vi "Write ItemID.vi"(8 "error in (no error)":errorcluster, 10 "ItemID":string, 11 "Standard VI Type in":refnum<class "Standard VI Type.lvclass">) -> (0 "error out":errorcluster, 3 "Standard VI Type out":refnum<class "Standard VI Type.lvclass">)   [LabVIEW 2020]
doc: "Basic write acceessor."
uses:
  Standard VI Type.lvclass
  Standard VI Type.lvclass/Standard VI Type.ctl
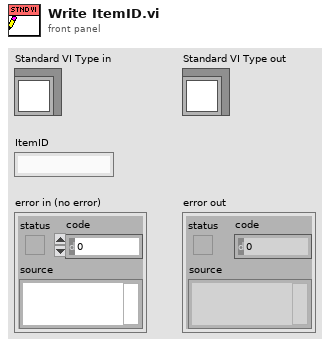
[diagram p1: front panel]
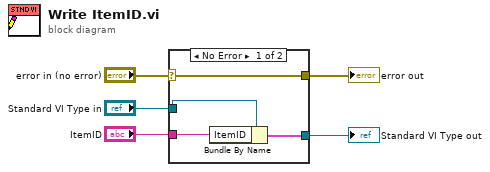
[diagram p0: block diagram]
diagram:
  n1 = case shown="No Error" "error in (no error)" {
    selector: "error in (no error)" -> [w9 w10]
    tunnel: [w9 w10] -> w4
    tunnel: [w7 w11] -> w2
    tunnel: "Standard VI Type in" -> [w8 w11]
    tunnel: "ItemID" -> [w6 _]
    frame No Error {
      n2 = Bundle By Name(cluster=w8, "ItemID"=w6) -> (w7:cluster{})
    }
    frame Error {
    }
  }
  "error out" <- w4
  "Standard VI Type out" <- w2
